vi "tt20_make_correlation.vi"(8 "error in (no error)":errorcluster, 10 "histo_settings":T1, 11 "tt20 in":refnum<class "tt20.lvclass">) -> (0 "error out":errorcluster, 3 "tt20 out":refnum<class "tt20.lvclass">)   [LabVIEW 2015, in "tt20.lvclass"]
uses:
  tt20.lvclass
  tt20_histo_settings_tdef.ctl
  tt20.lvclass/tt20.ctl
  C:/Users/MX-Microscope/Documents/LabVIEW Data/lvoop_campus_2018/Detector_Class/Swabian/time_tagger_vis/TTCSharp32.dll
  time_tagger_vis/TTCSharp32.dll
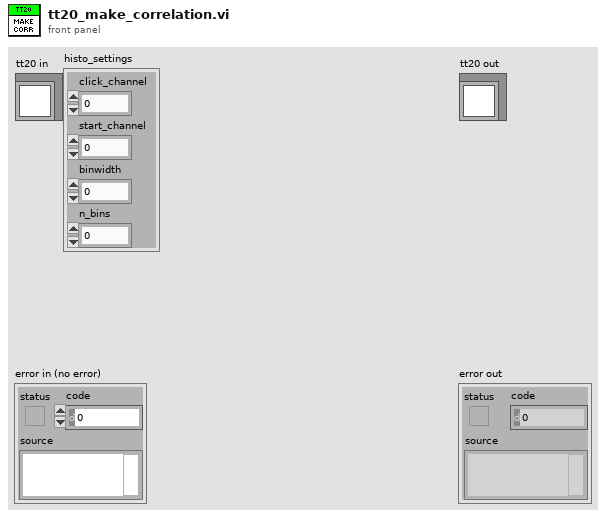
[diagram p1: front panel]
types:
  T1 = typedef "tt20_histo_settings_tdef.ctl" = cluster{"click_channel":u32, "start_channel":u32, "binwidth":i64, "n_bins":i32}
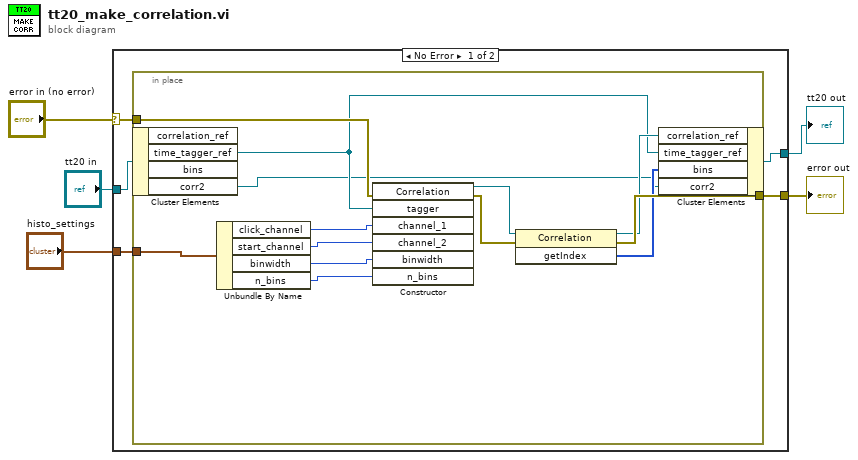
[diagram p0: block diagram]
diagram:
  n1 = case shown="No Error" "error in (no error)" {
    selector: "error in (no error)" -> [w10 w25]
    tunnel: [w9 w25] -> w4
    tunnel: [w6 w24] -> w2
    tunnel: "tt20 in" -> [w7 w24]
    tunnel: "histo_settings" -> [w8 _]
    frame No Error {
      n2 = in-place {
        in-place-border: w10 -> [w23]
        in-place-border: [w19] -> w9
        in-place-border: w8 -> [w22]
        n3 = in-place-cluster #1(w7) -> ("time_tagger_ref"=w16:refnum<k24>, "corr2"=w11:refnum<k24>)  [unwired: 2 out]
        n4 = Unbundle By Name(w22) -> ("click_channel"=w15:u32, "start_channel"=w14:u32, "binwidth"=w13:i64, "n_bins"=w12:i32)
        n5 = constructor class="Correlation"(error in=w23, "tagger"=w16, "channel_1"=w15, "channel_2"=w14, "binwidth"=w13, "n_bins"=w12) -> (reference out=w21:refnum<k24>, error out=w20:errorcluster)  [unwired: 2 in, 6 out]
        n6 = invoke class="Correlation" method="getIndex"(reference=w21, error in=w20) -> (reference out=w17:refnum<k24>, error out=w19:errorcluster, "getIndex"=w18:i64[])  [unwired: 1 in]
        n7 = in-place-cluster #1("correlation_ref"=w17, "time_tagger_ref"=w16, "bins"=w18, "corr2"=w11) -> (w6:refnum<class "tt20.lvclass">)
      }
    }
    frame Error {
    }
  }
  "error out" <- w4
  "tt20 out" <- w2
